vi "Initialize.vi"(8 "error in (no error)":errorcluster, 10 "eventLogDirectory":path) -> (0 "error out":errorcluster, 3 "EventFile out":refnum<class "EventFile.lvclass">)   [LabVIEW 2016, in "Event Logging.lvlib" / "EventFile.lvclass"]
uses:
  EventFile.lvclass
  EventFile.lvclass/EventFile.ctl
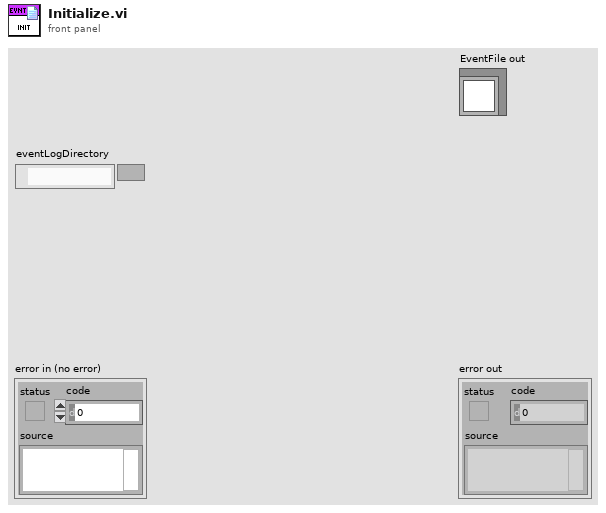
[diagram p1: front panel]
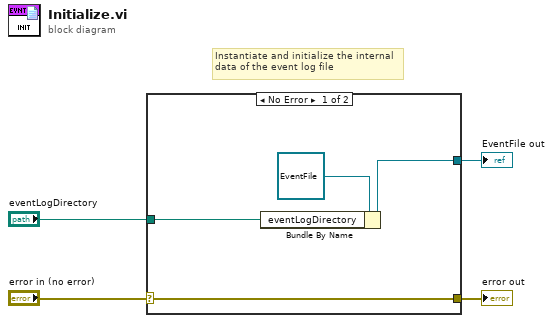
[diagram p0: block diagram]
diagram:
  # "Instantiate and initialize the internal\ndata of the event log file"
  n1 = case shown="No Error" "error in (no error)" {
    selector: "error in (no error)" -> [w8 w9]
    tunnel: [w8 w9] -> w3
    tunnel: [w6 _] -> w2
    tunnel: "eventLogDirectory" -> [w5 _]
    frame No Error {
      n2 = Bundle By Name(cluster=refnum<class "EventFile.lvclass"> refnum ("EventFile in"), "eventLogDirectory"=w5) -> (w6:refnum<class "EventFile.lvclass">)
    }
    frame Error {
    }
  }
  "error out" <- w3
  "EventFile out" <- w2
